vi "FTW-ActorRef-SpawnNewActor.vi"(0 "Actor Ref Prototype":refnum<class "FTW-EventLogger-API.lvclass">, 11 "error in":errorcluster) -> (4 "Actor Reference":refnum<class "FTW-EventLogger-API.lvclass">, 15 "error out":errorcluster)   [LabVIEW 2013, in "FTW-EventLogger-API.lvclass"]
uses:
  FTW-EventLogger-API.lvclass
panel:
  # "Inputs"
  # "Outputs"
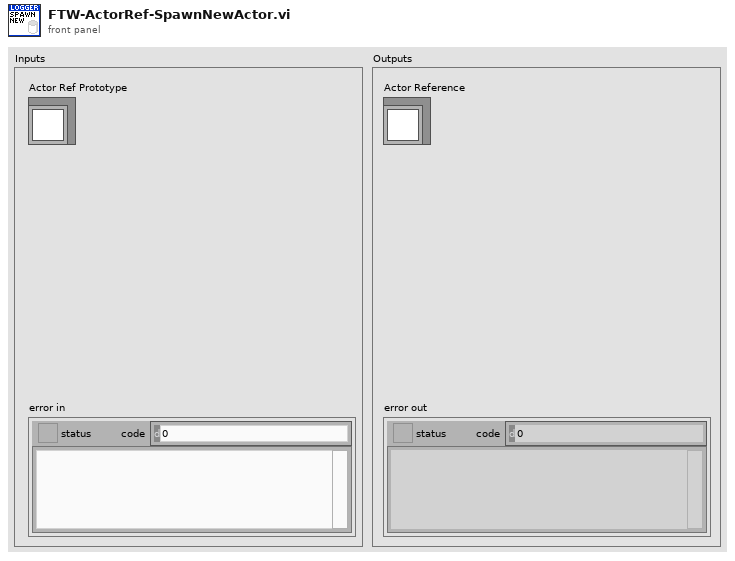
[diagram p1: front panel]
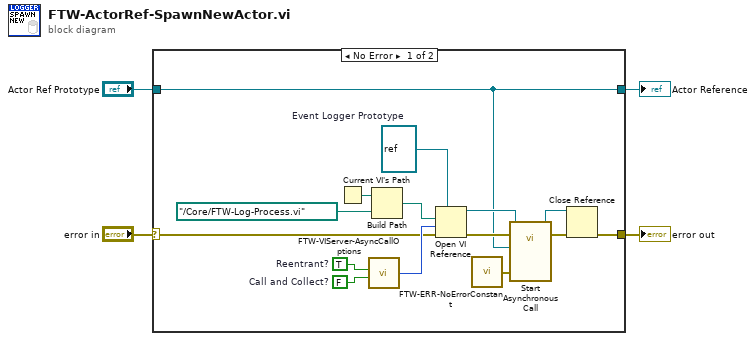
[diagram p0: block diagram]
diagram:
  n1 = case shown="No Error" "error in" {
    selector: "error in" -> [w6 w21]
    tunnel: "Actor Ref Prototype" -> [w5 w20]
    tunnel: [w5 w20] -> w4
    tunnel: [w16 w21] -> w3
    frame No Error {
      w15 = refnum<vi> refnum  # Event Logger Prototype
      w17 = FALSE  # Call and Collect?
      w18 = TRUE  # Reentrant?
      n2 = Current VI's Path() -> (path=w8:path)
      n3 = call "FTW-VIServer-AsyncCallOptions.vi"("Call and Collect?"=w17, "Reentrant?"=w18) -> ("Open VI Ref Options"=w19:i32)  [unwired: 4 in]
      n4 = Build Path(base path=w8, name or relative path=path "../Core/FTW-Log-Process.vi") -> (appended path=w7:path)
      n5 = Open VI Reference(type specifier VI Refnum (for type only)=w15, vi path=w7, options=w19, error in (no error)=w6) -> (vi reference=w14:refnum<vi>, error out=w13:errorcluster)  [unwired: 2 in]
      n6 = call "FTW-ERR-NoErrorConstant.vi"() -> ("no error"=w12:errorcluster)
      n7 = call-by-ref "Start Asynchronous Call"(reference=w14, error in=w13, "Event Logger API"=w5, "error in"=w12) -> (reference out=w11:refnum<vi>, error out=w10:errorcluster)  [unwired: 13 in, 1 out]
      n8 = Close Reference(reference=w11, error in (no error)=w10) -> (error out=w16:errorcluster)
    }
    frame Error {
    }
  }
  "error out" <- w3
  "Actor Reference" <- w4
